vi "2D Picture.vi"(6 "colors":u32[](array[colorbox])=[0, 10735, 16717824, 6422361], 7 "position array":dbl[][](array[numeric]), 9 "scale":cluster{"x":dbl, "y":dbl}={"x"=100.0, "y"=-100.0}, 10 "Origin":cluster{"x":dbl, "y":dbl}={"x"=100.0, "y"=200.0}, 11 "picture in":picture) -> (3 "picture out":picture)   [LabVIEW 2024]
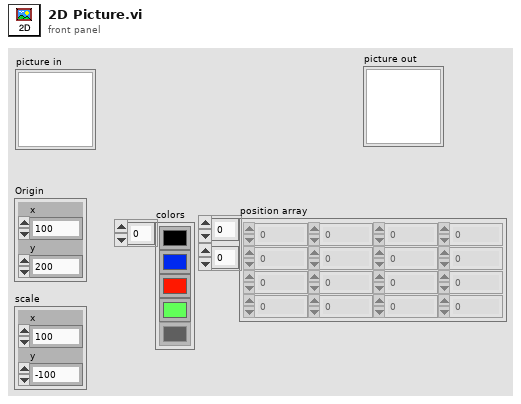
[diagram p1: front panel]
types:
  T1 = cluster{"Real Matrix Element":dbl, "Real Matrix Element":dbl}
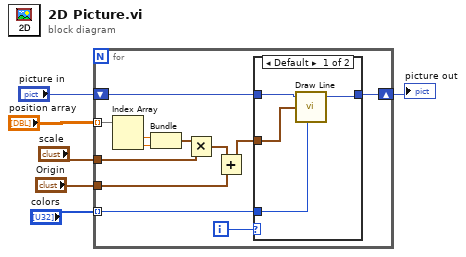
[diagram p0: block diagram]
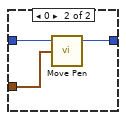
[diagram p2: hidden frame]
diagram:
  n1 = for {
    tunnel: "position array" -> [w14] mode=indexing
    shift-right: [w17] -> w4
    shift-left: "picture in" -> [w13]
    tunnel: "Origin" -> [w12]
    tunnel: "scale" -> [w10]
    tunnel: "colors" -> [w8] mode=indexing
    i -> [w18]
    n2 = Index Array(array=w14) -> (element #1=w16:dbl, element #2=w15:dbl)  [unwired: 2 in]
    n3 = Bundle("Real Matrix Element"=w16, "Real Matrix Element"=w15) -> (w11:T1)  [unwired: 1 in]
    n4 = Multiply(x=w11, y=w10) -> (x*y=w9:cluster{dbl, dbl})
    n5 = Add(x=w9, y=w12) -> (x+y=w7:cluster{dbl, dbl})
    n6 = case shown="Default" w18 {
      tunnel: [w22 w25] -> w17
      tunnel: w7 -> [w20 w24]
      tunnel: w13 -> [w21 w23]
      tunnel: w8 -> [w19 _]
      frame Default {
        n7 = call <vilib>:"Draw Line.vi"("picture"=w21, "end point"=w20, "color(black)"=w19) -> ("new picture"=w22:picture)  [unwired: 6 in]
      }
      frame 0 {
        n8 = call <vilib>:"Move Pen.vi"("new position"=w24, "picture"=w23) -> ("new picture"=w25:picture)  [unwired: 3 in]
      }
    }
  }
  "picture out" <- w4
